vi "Handle Pending Focus Update.vi"(6 "Time":u32, 8 "error in (no error)":errorcluster, 11 "App in":refnum<class "App.lvclass">) -> (0 "error out":errorcluster, 3 "App out":refnum<class "App.lvclass">)   [LabVIEW 2020, in "AR Example.lvlib" / "App.lvclass"]
uses:
  App.lvclass
  App.lvclass/App.ctl
  g_ar_toolkit.capture/CameraStream/CameraStream.lvclass/CameraStream.ctl
  g_ar_toolkit.capture/CameraStream/Set Focus Parameter.vi
  g_ar_toolkit.capture/CameraStream/SetParameter.vi
  g_ar_toolkit.common/Module Path.vi
  <vilib>/Utility/error.llb/Error Cluster From Error Code.vi
  g_ar_toolkit.capture/CameraStream/CameraStream.lvclass
  UI/UI.lvclass
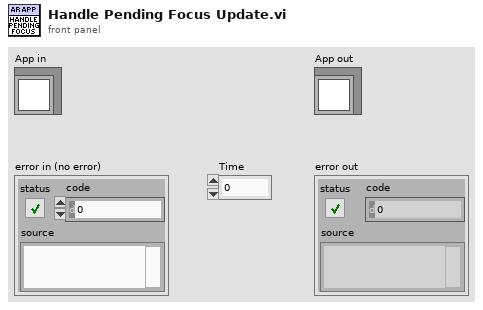
[diagram p1: front panel]
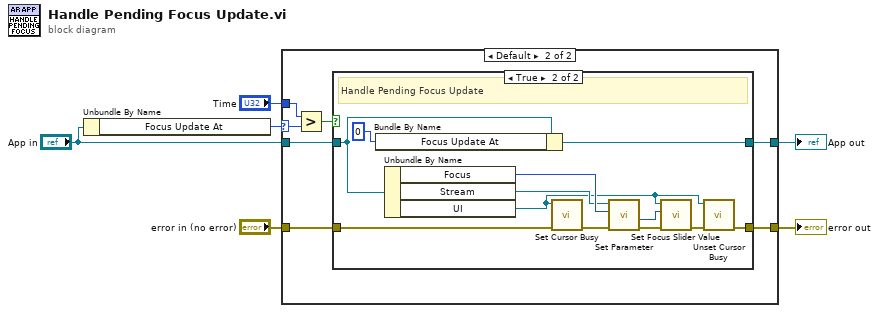
[diagram p0: block diagram]
diagram:
  n1 = Unbundle By Name("App in") -> ("Focus Update At"=w2:u32)
  n2 = case shown="Default" w2 {
    selector: w2 -> [_ w10]
    tunnel: [w8 w15] -> w6
    tunnel: [w7 w14] -> w5
    tunnel: "error in (no error)" -> [w8 w13]
    tunnel: "App in" -> [w7 w12]
    tunnel: "Time" -> [_ w11]
    frame 0 {
    }
    frame Default {
      n3 = Greater?(x=w11, y=w10) -> (0:w9:bool)
      n4 = case shown="True" w9 {
        tunnel: w13 -> [w16 w28]
        tunnel: w12 -> [w17 w27]
        tunnel: [w17 w22] -> w14
        tunnel: [w16 w25] -> w15
        frame False {
        }
        frame True {
          # "Handle Pending Focus Update"
          n5 = Bundle By Name(cluster=w27, "Focus Update At"=u32 0 ("Camera Setup.Focus Update At")) -> (w22:refnum<class "App.lvclass">)
          n6 = Unbundle By Name(w27) -> ("Focus"=w26:i32, "Stream"=w23:refnum<class "CameraStream.lvclass">, "UI"=w19:refnum<class "UI.lvclass">)
          n7 = call "Set Cursor Busy.vi"("error in (no error)"=w28, "UI in"=w19) -> ("error out"=w29:errorcluster)  [unwired: 9 in]
          n8 = call-poly "Set Parameter.vi"("error in (no error)"=w29, "Value"=w26, "CameraStream in"=w23) -> ("error out"=w24:errorcluster, "Set Value"=w18:i32)  [unwired: 6 in, 1 out]
          n9 = call "Set Focus Slider Value.vi"("error in (no error)"=w24, "Value"=w18, "UI in"=w19) -> ("error out"=w20:errorcluster)  [unwired: 8 in]
          n10 = call "Unset Cursor Busy.vi"("error in (no error)"=w20, "UI in"=w19) -> ("error out"=w25:errorcluster)  [unwired: 9 in]
        }
      }
    }
  }
  "error out" <- w6
  "App out" <- w5
